vi "create.vi"(4 "Default Headers":T1[](array[typedef]), 5 "Client type":refnum<class "Client.lvclass">, 6 "Verify Server(true)":bool=TRUE, 8 "error in (no error)":errorcluster) -> (0 "error out":errorcluster, 3 "Client out":refnum<class "Client.lvclass">)   [LabVIEW 2020, in "reqwest.lvlib" / "Client.lvclass"]
uses:
  Client.lvclass
  Client.lvclass/Client.ctl
  ClientBuilder/ClientBuilder.lvclass
  Headers/Headers.lvclass
  <vilib>/addons/_JKI.lib/REST Client/classes/REST Client/HTTP Header.ctl
  <vilib>/addons/_JKI.lib/REST Client/classes/REST Client/REST Client.lvclass
panel:
  in  "connect_timeout_secs":u64
  in  "timeout_secs":u64
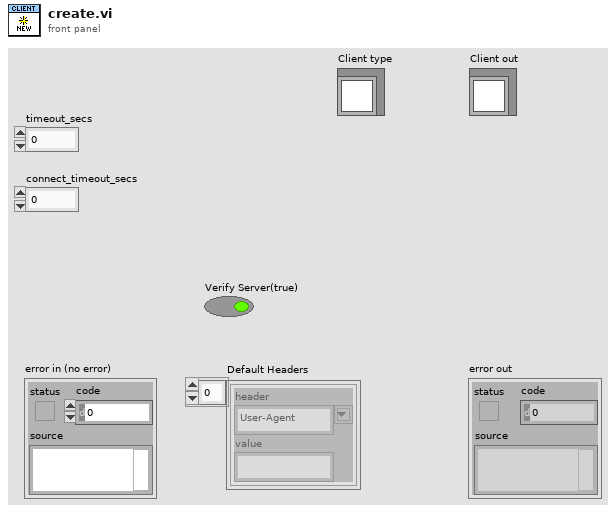
[diagram p1: front panel]
types:
  T1 = typedef "REST Client.lvlib/REST Client.lvclass/HTTP Header.ctl" = cluster{"header":string, "value":string}
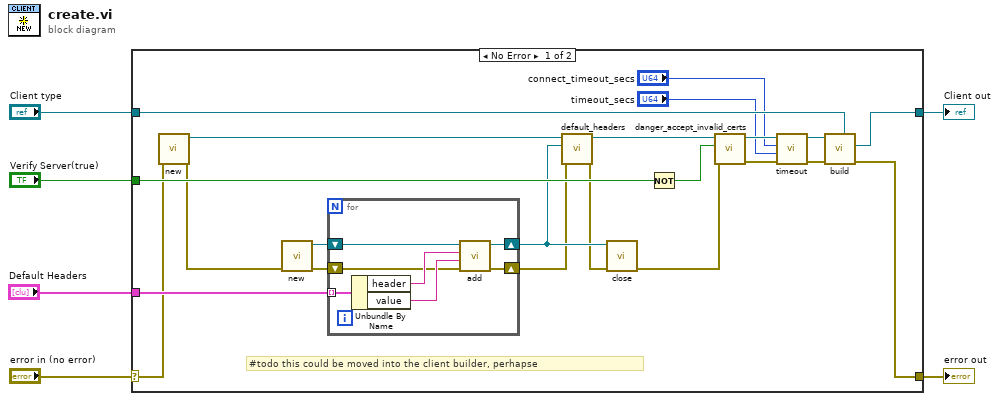
[diagram p0: block diagram]
diagram:
  n1 = case shown="No Error" "error in (no error)" {
    selector: "error in (no error)" -> [w15 w37]
    tunnel: [w13 w37] -> w5
    tunnel: [w20 w36] -> w3
    tunnel: "Client type" -> [w19 w36]
    tunnel: "Default Headers" -> [w28 _]
    tunnel: "Verify Server(true)" -> [w25 _]
    frame No Error {
      # "#todo this could be moved into the client builder, perhapse"
      n2 = call "new.vi"("error in (no error)"=w15) -> ("error out"=w14:errorcluster, "Client out"=w23:refnum<class "ClientBuilder.lvclass">)  [unwired: 9 in]
      n3 = call "new.vi"("error in (no error)"=w14) -> ("error out"=w26:errorcluster, "Headers out"=w27:refnum<class "Headers.lvclass">)  [unwired: 9 in]
      n4 = for {
        tunnel: w28 -> [w33] mode=indexing
        shift-right: [w35] -> w21
        shift-left: w27 -> [w34]
        shift-right: [w29] -> w16
        shift-left: w26 -> [w30]
        n5 = Unbundle By Name(w33) -> ("header"=w32:string, "value"=w31:string)
        n6 = call "add.vi"("error in (no error)"=w30, "value"=w31, "key"=w32, "Headers in"=w34) -> ("error out"=w29:errorcluster, "Headers out"=w35:refnum<class "Headers.lvclass">)  [unwired: 5 in, 1 out]
      }
      n7 = call "default_headers.vi"("error in (no error)"=w16, "Headers"=w21, "ClientBuilder in"=w23) -> ("error out"=w18:errorcluster, "ClientBuilder out"=w22:refnum<class "ClientBuilder.lvclass">)  [unwired: 6 in, 1 out]
      n8 = call "close.vi"("error in (no error)"=w18, "Headers in"=w21) -> ("error out"=w17:errorcluster)  [unwired: 9 in]
      n9 = Not(x=w25) -> (.not. x?=w24:bool)
      n10 = call "danger_accept_invalid_certs.vi"("error in (no error)"=w17, "danger_accept_invalid_certs"=w24, "ClientBuilder in"=w22) -> ("error out"=w10:errorcluster, "ClientBuilder out"=w12:refnum<class "ClientBuilder.lvclass">)  [unwired: 6 in, 1 out]
      n11 = call "timeout.vi"("error in (no error)"=w10, "timeout_secs"="timeout_secs", "connect_timeout_secs"="connect_timeout_secs", "ClientBuilder in"=w12) -> ("error out"=w9:errorcluster, "ClientBuilder out"=w11:refnum<class "ClientBuilder.lvclass">)  [unwired: 5 in, 1 out]
      n12 = call "build.vi"("Client type"=w19, "error in (no error)"=w9, "ClientBuilder in"=w11) -> ("error out"=w13:errorcluster, "Client out"=w20:refnum<class "Client.lvclass">)  [unwired: 7 in]
    }
    frame Error {
    }
  }
  "error out" <- w5
  "Client out" <- w3
